vi "WAM_BarCode_PopupWithPhoto.vi"(0 "Enable":bool=TRUE, 5 "error in (no error)":errorcluster) -> (14 "msn":string, 17 "Bar Code":string, 18 "OK":bool, 19 "error out":errorcluster)   [LabVIEW 2018]
doc: "Displays a standard dialog box that prompts users to enter information, such as a user name and password.\n--------------------\n\nThis Express VI is configured as follows:\n\nMessage to Display to the User:Scan the WAM Barcode,\nThe bar code is located on the top of the WAM module\nThe inputs are: \nText Entry Box: Bar Code"
panel:
  in  "Bar Code":string
  out "String":string="Scan the WAM Barcode,\nThe bar code is located on the top of the WAM module"
  in  "Cancel":bool
  in  "OK2":bool
  in  "OK1":bool
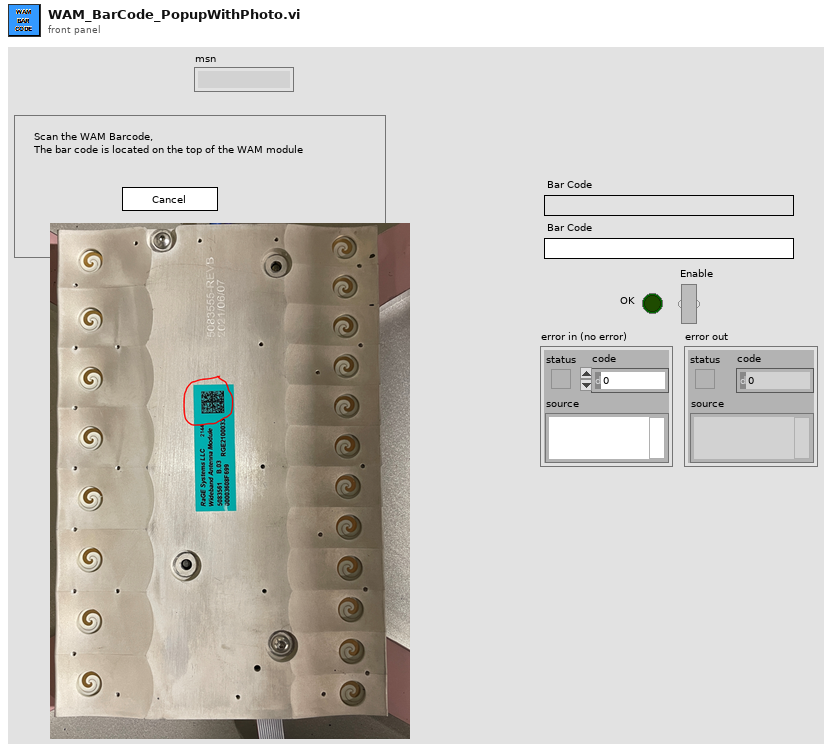
[diagram p1: front panel]
types:
  T1 = cluster{"Input Name":string, "Input Data Type":i32}[]
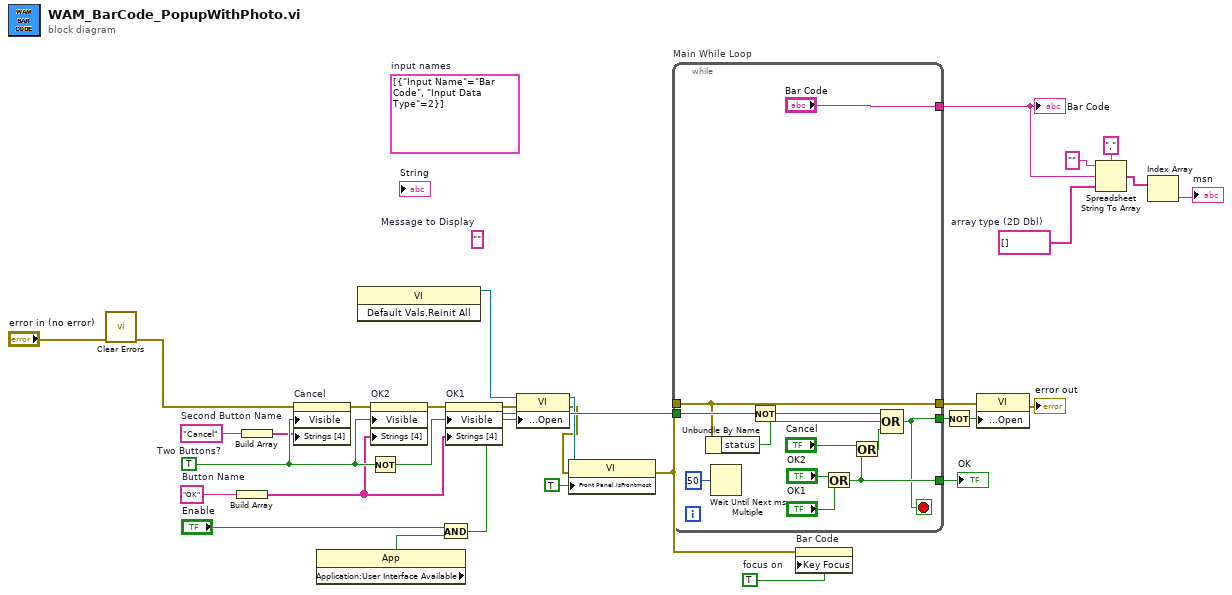
[diagram p0: block diagram]
diagram:
  w5 = string[] []  # array type (2D Dbl)
  w12 = TRUE  # focus on
  (unwired) T1 [{"Input Name"="Bar Code", "Input Data Type"=2}]  # input names
  w23 = "Cancel"  # Second Button Name
  w21 = "OK"  # Button Name
  (unwired) ""  # Message to Display
  w31 = TRUE  # Two Buttons?
  n1 = call <vilib>:"Clear Errors.vi"("error in (no error)"="error in (no error)") -> ("error out"=w7:errorcluster)  [unwired: 5 in, 1 out]
  n2 = Build Array(w21) -> (w22:string[])
  n3 = Build Array(w23) -> (w24:string[])
  n4 = property on="Cancel" class="Bool"(error in=w7, "Visible"=w31, "Strings [4]"=w24) -> (error out=w28:errorcluster)  [unwired: 1 in, 1 out]
  n5 = property class="App"() -> ("Application:User Interface Available"=w14:bool)  [unwired: 2 in, 2 out]
  n6 = invoke class="VI" method="Default Vals.Reinit All"() -> (reference out=w13:refnum<vi>)  [unwired: 3 in, 2 out]
  n7 = Not(x=w31) -> (.not. x?=w29:bool)
  n8 = property on="OK2" class="Bool"(error in=w28, "Visible"=w31, "Strings [4]"=w22) -> (error out=w27:errorcluster)  [unwired: 1 in, 1 out]
  n9 = And(x="Enable", y=w14) -> (x .and. y?=w15:bool)
  n10 = property on="OK1" class="Bool"(error in=w27, "Visible"=w29, "Strings [4]"=w22) -> (error out=w20:errorcluster)  [unwired: 1 in, 1 out]
  n11 = property class="VI"(reference=w13, error in=w20, "Front Panel Window:Open"=w15) -> (reference out=w11:refnum<vi>, error out=w10:errorcluster)
  n12 = property class="VI"(reference=w11, error in=w10, "Front Panel.IsFrontmost"=TRUE ("Front Panel Window:Is Frontmost")) -> (error out=w9:errorcluster)  [unwired: 1 out]
  n13 = while "Main While Loop" {
    tunnel: [w40] -> w30
    tunnel: w15 -> [w38]
    tunnel: [w36] -> w25
    tunnel: w9 -> [w35]
    tunnel: [w35] -> w18
    tunnel: ["Bar Code"] -> w6
    stop <- w36 stop-if-true
    n14 = Unbundle By Name(w35) -> ("status"=w33:bool)
    n15 = Wait Until Next ms Multiple(millisecond multiple=u32 50) -> ()  [unwired: 1 out]
    n16 = Not(x=w38) -> (.not. x?=w37:bool)
    n17 = Or(x="OK2", y="OK1") -> (x .or. y?=w40:bool)
    n18 = Or(x="Cancel", y=w40) -> (x .or. y?=w34:bool)
    n19 = Compound Arithmetic op=OR(w37, w33, w34) -> (w36:bool)
  }
  "OK" <- w30
  "Bar Code" <- w6
  n20 = property on="Bar Code" class="Str"(error in=w9, "Key Focus"=w12) -> ()  [unwired: 1 in, 2 out]
  n21 = Not(x=w25) -> (.not. x?=w26:bool)
  n22 = property class="VI"(error in=w18, "Front Panel Window:Open"=w26) -> (error out=→"error out":errorcluster)  [unwired: 1 in, 1 out]
  n23 = Spreadsheet String To Array(delimiter (Tab)=",", format string="", spreadsheet string=w6, array type (2D Dbl)=w5) -> (array=w4:string[])
  n24 = Index Array(array=w4) -> (element=→"msn":string)  [unwired: 1 in]
